vi "Read offset.vi"(8 "error in (no error)":errorcluster, 11 "Configuration.Channel in":refnum<class "Configuration.Channel.lvclass">) -> (0 "error out":errorcluster, 2 "offset":u64, 3 "Configuration.Channel out":refnum<class "Configuration.Channel.lvclass">)   [LabVIEW 2016, in "Configuration.Channel.lvclass"]
uses:
  Configuration.Channel.lvclass
  Configuration.Channel.lvclass/Configuration.Channel.ctl
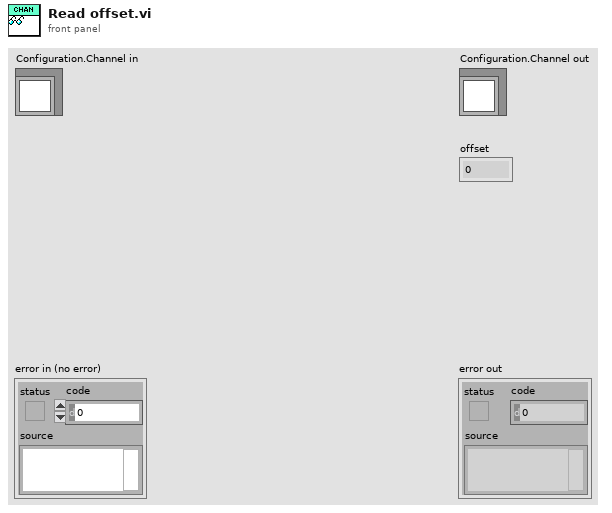
[diagram p1: front panel]
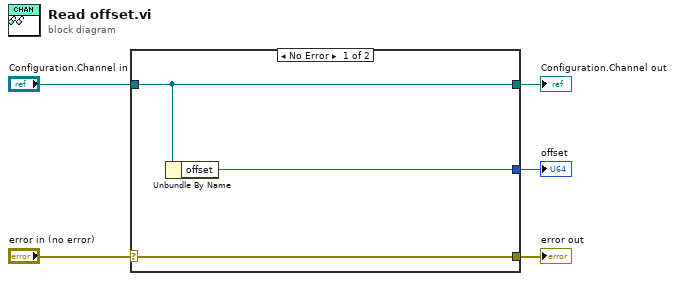
[diagram p0: block diagram]
diagram:
  n1 = case shown="No Error" "error in (no error)" {
    selector: "error in (no error)" -> [w8 w9]
    tunnel: [w8 w9] -> w4
    tunnel: [w7 w10] -> w2
    tunnel: "Configuration.Channel in" -> [w7 w10]
    tunnel: [w6 _] -> w1
    frame No Error {
      n2 = Unbundle By Name(w7) -> ("offset"=w6:u64)
    }
    frame Error {
    }
  }
  "error out" <- w4
  "Configuration.Channel out" <- w2
  "offset" <- w1
